vi "Parse Comments and Commands.vi"(3 "ITX Notes and Commands":string) -> (0 "Commands":string, 1 "Notes":string)   [LabVIEW 2019, in "Data.ITX.lvclass"]
uses:
  Data.ITX.lvclass
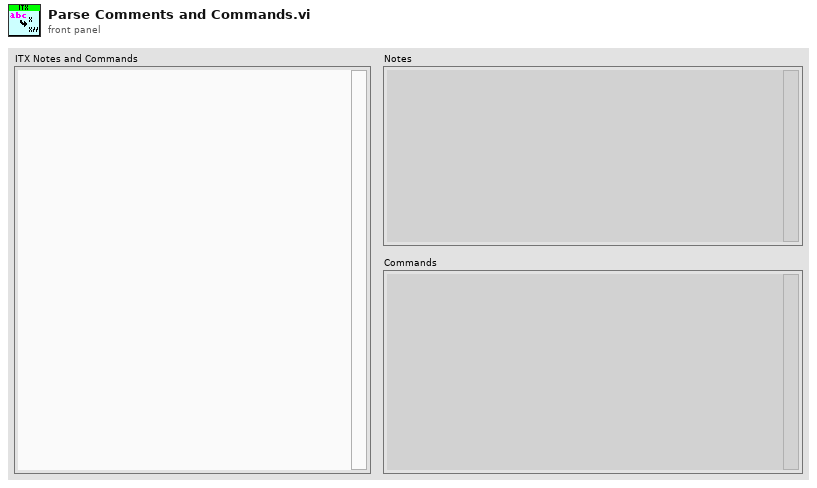
[diagram p1: front panel]
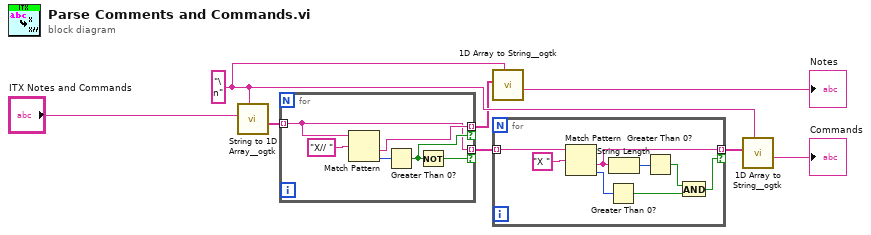
[diagram p0: block diagram]
diagram:
  w5 = "\n" ("delimiter (Tab)")
  n1 = call "String to 1D Array__ogtk.vi"("delimiter (Tab)"=w5, "string"="ITX Notes and Commands") -> ("Array of Strings"=w1:string[])  [unwired: 9 in]
  n2 = for {
    tunnel: w1 -> [w9] mode=indexing
    tunnel: [w12] -> w3 mode=indexing if=w10
    tunnel: [w9] -> w2 mode=indexing if=w14
    n3 = Match Pattern(string=w9, regular expression="X// " ("String")) -> (after substring=w12:string, offset past match=w11:i32)  [unwired: 3 out]
    n4 = Greater Than 0?(x=w11) -> (x > 0?=w10:bool)
    n5 = Not(x=w10) -> (.not. x?=w14:bool)
  }
  n6 = call "1D Array to String__ogtk.vi"("delimiter (Tab)"=w5, "Array of Strings"=w3) -> ("delimited string"=→"Notes":string)  [unwired: 9 in]
  n7 = for {
    tunnel: w2 -> [w21] mode=indexing
    tunnel: [w19] -> w4 mode=indexing if=w15
    n8 = Match Pattern(string=w21, regular expression="X " ("String")) -> (after substring=w19:string, offset past match=w20:i32)  [unwired: 3 out]
    n9 = Greater Than 0?(x=w20) -> (x > 0?=w16:bool)
    n10 = String Length(string=w19) -> (length=w18:i32)
    n11 = Greater Than 0?(x=w18) -> (x > 0?=w17:bool)
    n12 = And(x=w17, y=w16) -> (x .and. y?=w15:bool)
  }
  n13 = call "1D Array to String__ogtk.vi"("delimiter (Tab)"=w5, "Array of Strings"=w4) -> ("delimited string"=→"Commands":string)  [unwired: 9 in]
